vi "Refresh Display.vi"(8 "error in":errorcluster, 11 "Fault Handler in":refnum<class "Fault Handler.lvclass">) -> (0 "error out":errorcluster, 3 "Fault Handler out":refnum<class "Fault Handler.lvclass">)   [LabVIEW 2023, in "Fault Handler.lvlib" / "Fault Handler.lvclass"]
doc: "This routine uses the error and system state to determine if there is a state transition and if so, how to act on the state transition.\n\nIf only a warning is present, the software makes the entire panel Yellow\nIf no error is present, the software makes the entire panel the default color.\nIf an error is present, the software makes the entire panel Red\n Transmits a toggle component display == TRUE command (showing the display)\n\nFinally the software calls <b>Update System State</b>"
uses:
  Library/Fault Handler.lvclass
  C:/Users/Public/Documents/Development/builds/Engine/Engine.lvlibp/Project/Engine.lvclass
  Library/Fault Handler.lvclass/Fault Handler.ctl
  builds/Engine/Engine.lvlibp/Accessors/Read VI_Ref.vi
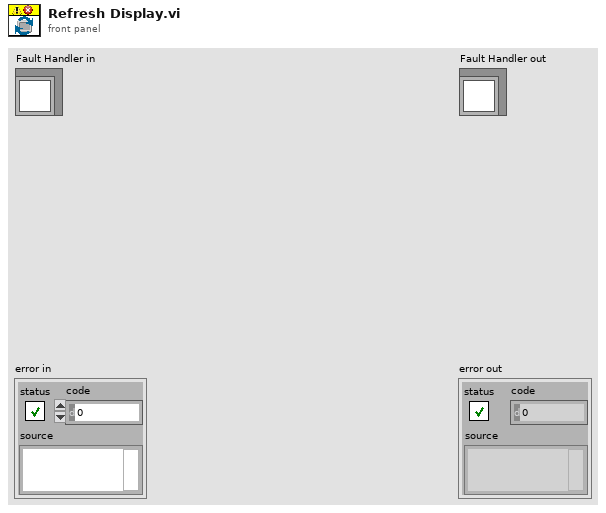
[diagram p1: front panel]
types:
  T1 = typedef "Engine.lvlibp/Engine.lvclass/System Status.ctl" = enum16{"Logged Off", "UUT_Info_Missing", "Idle", "Error", "Warning", "Loading", "Config", "Manual", "Automation", "Report_View", "Previous"}
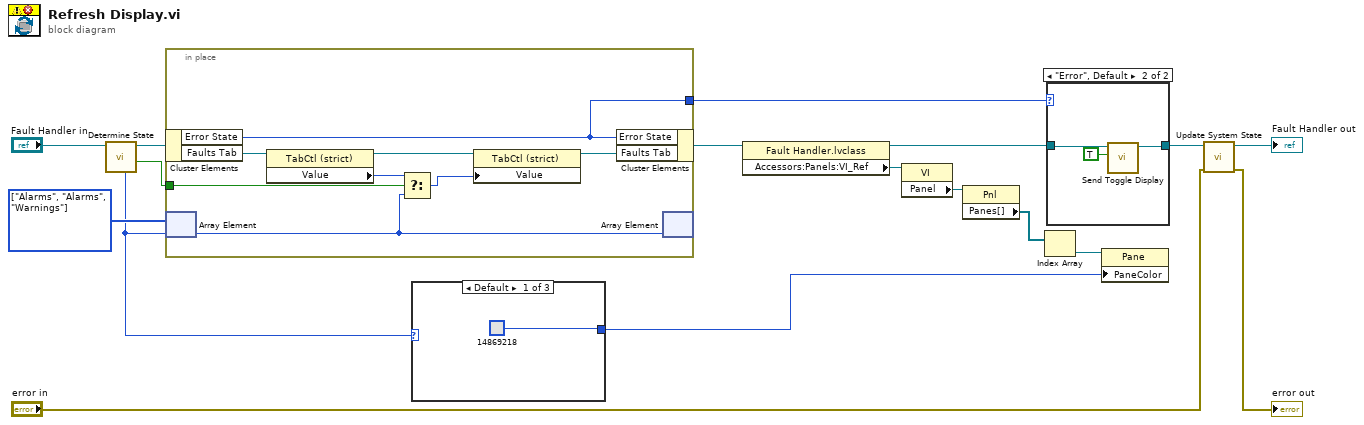
[diagram p0: block diagram]
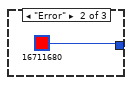
[diagram p2: hidden frame]
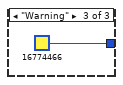
[diagram p3: hidden frame]
diagram:
  w12 = enum32{"Alarms", "Warnings"}[] [enum."Alarms", enum."Alarms", enum."Warnings"] items=["Alarms", "Warnings"]
  n1 = call "Determine State.vi"("Fault Handler in"="Fault Handler in") -> ("Nominal"=w3:bool, "Fault Handler out"=w10:refnum<class "Fault Handler.lvclass">, "Error State"=w2:T1)  [unwired: 7 in, 1 out]
  n2 = in-place {
    in-place-border: [w24] -> w9
    in-place-border: w3 -> [w18]
    n3 = in-place-cluster #1(w10) -> ("Error State"=w24:T1, "Faults Tab"=w23:refnum<vi>)
    n4 = in-place-array #2(w12, w2) -> (w20:enum32{"Alarms", "Warnings"})
    n5 = property class="TabCtl (strict)"(reference=w23) -> (reference out=w22:refnum<vi>, "Value"=w21:enum32{"Alarms", "Warnings"})  [unwired: 1 in, 1 out]
    n6 = Select(t=w21, s=w18, f=w20) -> (s? t:f=w19:enum32{"Alarms", "Warnings"})
    n7 = property class="TabCtl (strict)"(reference=w22, "Value"=w19) -> (reference out=w25:refnum<vi>)  [unwired: 1 in, 1 out]
    n8 = in-place-cluster #1("Error State"=w24, "Faults Tab"=w25) -> (w13:refnum<class "Fault Handler.lvclass">)
    n9 = in-place-array #2(w20) -> ()  [unwired: 2 out]
  }
  n10 = case shown="Default" w2 {
    tunnel: [u32 14869218 ("Color Box") u32 16711680 ("Color Box") u32 16774466 ("Color Box")] -> w1
    frame Default {
    }
    frame "Error" {
    }
    frame "Warning" {
    }
  }
  n11 = property class="Fault Handler.lvclass"(reference=w13) -> (reference out=w8:refnum<class "Fault Handler.lvclass">, "Accessors:Panels:VI_Ref"=w14:refnum<vi>)  [unwired: 1 in, 1 out]
  n12 = property class="VI"(reference=w14) -> ("Panel"=w15:refnum<vi>)  [unwired: 1 in, 2 out]
  n13 = property class="Pnl"(reference=w15) -> ("Panes[]"=w16:refnum<vi>[])  [unwired: 1 in, 2 out]
  n14 = Index Array(array=w16) -> (element=w17:refnum<vi>)  [unwired: 1 in]
  n15 = case shown="\"Error\", Default" w9 {
    tunnel: w8 -> [w29 w32]
    tunnel: [w29 w31] -> w7
    frame "Logged Off" {
    }
    frame "Error", Default {
      n16 = call "Send Toggle Display.vi"("Show"=TRUE, "Fault Handler in"=w32) -> ("Fault Handler out"=w31:refnum<class "Fault Handler.lvclass">)  [unwired: 8 in, 1 out]
    }
  }
  n17 = property class="Pane"(reference=w17, "PaneColor"=w1) -> ()  [unwired: 1 in, 2 out]
  n18 = call "Update System State.vi"("error in"="error in", "Fault Handler in"=w7) -> ("error out"=→"error out":errorcluster, "Fault Handler out"=→"Fault Handler out":refnum<class "Fault Handler.lvclass">)  [unwired: 8 in]
